vi "HGF_DSCVarManagerTask.vi"(1 "Task Trigger":refnum<class>, 2 "Task Destination":refnum<class>, 3 "Task Exception Event":refnum<class>, 5 "error in (no error)":errorcluster, 8 "timeout in ms (10000)":i32=10000, 9 "object/ProcessName":string) -> (14 "VarManager TaskLoop":refnum<class "HGF_TaskLoop.lvclass">, 16 "Task Trigger Event":refnum<class "HGF_Event.lvclass">, 17 "Task Destination Event":refnum<class "HGF_Event.lvclass">, 18 "ExceptionTriggerEvent":refnum<class "HGF_TriggeredEvent.lvclass">, 19 "error out":errorcluster)   [LabVIEW 2012, in "HGF_DSC.lvlib" / "HGF_DSCVarManager.lvclass"]
uses:
  HGF_DSCVarManager.lvclass
  HGF_BaseClasses/HGF_TriggeredEvent/HGF_TriggeredEvent.lvclass
  HGF_BaseClasses/HGF_Event/HGF_Event.lvclass
  HGF_BaseClasses/HGF_TaskLoop/HGF_TaskLoop.lvclass
  HGF_DSCFactory/HGF_DSCFactory.lvclass
  HGF_BaseClasses/HGF_Notifier/HGF_Notifier.lvclass
  HGF_BaseClasses/HGF_TaskOnce/HGF_TaskOnce.lvclass
  HGF_BaseClasses/HGF_ThreadTask/HGF_ThreadTask.lvclass
  HGF_BaseClasses/HGF_Factory/HGF_Factory.lvclass
  HGF_BaseClasses/HGF_Queue/HGF_Queue.lvclass
  HGF_BaseClasses/HGF_Timing/HGF_Timing.lvclass
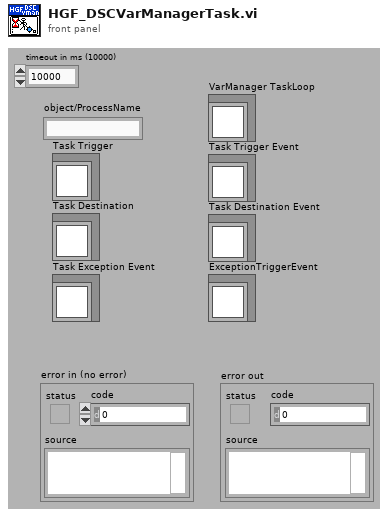
[diagram p1: front panel]
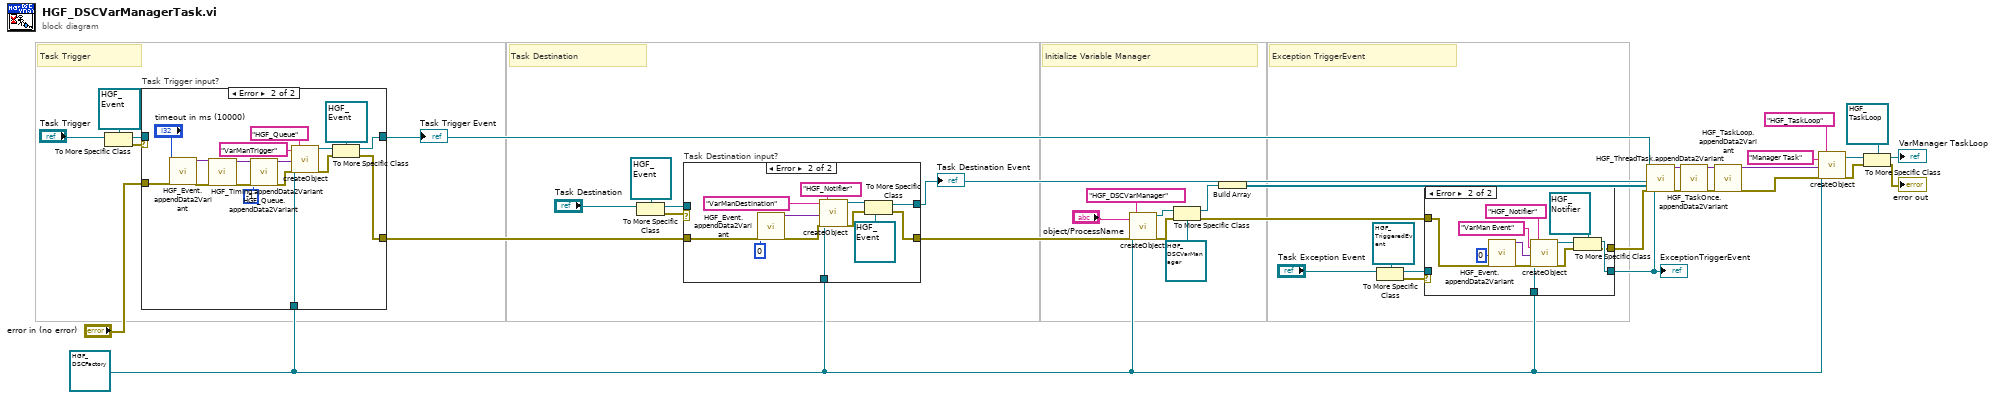
[diagram p0: block diagram]
diagram:
  w31 = refnum<class "HGF_DSCFactory.lvclass"> refnum ("DSC.lvlib:HGF_DSCFactory.lvclass")
  # "Exception TriggerEvent"
  # "Initialize Variable Manager"
  # "Task Destination"
  # "Task Trigger"
  n1 = To More Specific Class(target class=refnum<class "HGF_Event.lvclass"> refnum ("HGF_BaseClasses.lvlib:HGF_Event.lvclass"), reference="Task Trigger") -> (specific class reference=w29:refnum<class "HGF_Event.lvclass">, error out=w28:errorcluster)  [unwired: 1 in]
  n2 = case "Task Trigger input?" shown="Error" w28 {
    tunnel: w31 -> [_ w60]
    tunnel: [w43 w57] -> w30
    tunnel: [w42 w48] -> w35
    tunnel: "error in (no error)" -> [w42 w47]
    tunnel: w29 -> [w43 _]
    frame No Error {
    }
    frame Error {
      n3 = call "HGF_Event.appendData2Variant.vi"("timeout in ms (-1)"="timeout in ms (10000)", "error in (no error)"=w47) -> ("dup initData"=w50:variant, "error out"=w49:errorcluster)  [unwired: 16 in]
      n4 = call "HGF_Timing.appendData2Variant.vi"("initData"=w50, "error in (no error)"=w49) -> ("dup initData"=w53:variant, "error out"=w52:errorcluster)  [unwired: 16 in]
      n5 = call "HGF_Queue.appendData2Variant.vi"("initData"=w53, "maxQueueSize (-1)"=-1, "error in (no error)"=w52) -> ("dup initData"=w56:variant, "error out"=w55:errorcluster)  [unwired: 15 in]
      n6 = call "createObject.vi"("HGF_Factory"=w60, "objectName"="VarManTrigger", "initializationData"=w56, "error in (no error)"=w55, "className"="HGF_Queue") -> ("HGF_Object"=w59:refnum<class "HGF_Factory.lvclass">, "error out"=w58:errorcluster)  [unwired: 12 in, 1 out]
      n7 = To More Specific Class(target class=refnum<class "HGF_Event.lvclass"> refnum ("HGF_BaseClasses.lvlib:HGF_Event.lvclass"), reference=w59, error in=w58) -> (specific class reference=w57:refnum<class "HGF_Event.lvclass">, error out=w48:errorcluster)
    }
  }
  "Task Trigger Event" <- w30
  n8 = To More Specific Class(target class=refnum<class "HGF_Event.lvclass"> refnum ("HGF_BaseClasses.lvlib:HGF_Event.lvclass"), reference="Task Destination") -> (specific class reference=w36:refnum<class "HGF_Event.lvclass">, error out=w34:errorcluster)  [unwired: 1 in]
  n9 = case "Task Destination input?" shown="Error" w34 {
    tunnel: [w62 w71] -> w16
    tunnel: [w61 w70] -> w3
    tunnel: w35 -> [w61 w67]
    tunnel: w31 -> [_ w64]
    tunnel: w36 -> [w62 _]
    frame No Error {
    }
    frame Error {
      n10 = call "HGF_Event.appendData2Variant.vi"("timeout in ms (-1)"=0, "error in (no error)"=w67) -> ("dup initData"=w69:variant, "error out"=w68:errorcluster)  [unwired: 16 in]
      n11 = call "createObject.vi"("HGF_Factory"=w64, "objectName"="VarManDestination", "initializationData"=w69, "error in (no error)"=w68, "className"="HGF_Notifier") -> ("HGF_Object"=w73:refnum<class "HGF_Factory.lvclass">, "error out"=w72:errorcluster)  [unwired: 12 in, 1 out]
      n12 = To More Specific Class(target class=refnum<class "HGF_Event.lvclass"> refnum ("HGF_BaseClasses.lvlib:HGF_Event.lvclass"), reference=w73, error in=w72) -> (specific class reference=w71:refnum<class "HGF_Event.lvclass">, error out=w70:errorcluster)
    }
  }
  "Task Destination Event" <- w16
  n13 = call "createObject.vi"("HGF_Factory"=w31, "objectName"="object/ProcessName", "error in (no error)"=w3, "className"="HGF_DSCVarManager") -> ("HGF_Object"=w13:refnum<class "HGF_Factory.lvclass">, "error out"=w15:errorcluster)  [unwired: 13 in, 1 out]
  n14 = To More Specific Class(target class=refnum<class "HGF_DSCVarManager.lvclass"> refnum ("DSC.lvlib:HGF_DSCVarManager.lvclass"), reference=w13, error in=w15) -> (specific class reference=w14:refnum<class "HGF_DSCVarManager.lvclass">, error out=w18:errorcluster)
  n15 = Build Array(w14) -> (w12:refnum<class "HGF_DSCVarManager.lvclass">[])
  n16 = To More Specific Class(target class=refnum<class "HGF_TriggeredEvent.lvclass"> refnum ("HGF_BaseClasses.lvlib:HGF_TriggeredEvent.lvclass"), reference="Task Exception Event") -> (specific class reference=w39:refnum<class "HGF_TriggeredEvent.lvclass">, error out=w38:errorcluster)  [unwired: 1 in]
  n17 = case shown="Error" w38 {
    tunnel: [w76 w84] -> w40
    tunnel: [w75 w83] -> w17
    tunnel: w18 -> [w75 w82]
    tunnel: w31 -> [_ w77]
    tunnel: w39 -> [w76 _]
    frame No Error {
    }
    frame Error {
      n18 = call "HGF_Event.appendData2Variant.vi"("timeout in ms (-1)"=0, "error in (no error)"=w82) -> ("dup initData"=w80:variant, "error out"=w81:errorcluster)  [unwired: 16 in]
      n19 = call "createObject.vi"("HGF_Factory"=w77, "objectName"="VarMan Event", "initializationData"=w80, "error in (no error)"=w81, "className"="HGF_Notifier") -> ("HGF_Object"=w87:refnum<class "HGF_Factory.lvclass">, "error out"=w86:errorcluster)  [unwired: 12 in, 1 out]
      n20 = To More Specific Class(target class=refnum<class "HGF_Notifier.lvclass"> refnum ("HGF_BaseClasses.lvlib:HGF_Notifier.lvclass"), reference=w87, error in=w86) -> (specific class reference=w84:refnum<class "HGF_Notifier.lvclass">, error out=w83:errorcluster)
    }
  }
  "ExceptionTriggerEvent" <- w40
  n21 = call "HGF_ThreadTask.appendData2Variant.vi"("taskTrigger"=w30, "taskDestination"=w16, "objectArray"=w12, "error in (no error)"=w17, "exceptionEvent"=w40) -> ("dup initData"=w4:variant, "error out"=w10:errorcluster)  [unwired: 13 in]
  n22 = call "HGF_TaskOnce.appendData2Variant.vi"("initData"=w4, "error in (no error)"=w10) -> ("dup initData"=w5:variant, "error out"=w9:errorcluster)  [unwired: 16 in]
  n23 = call "HGF_TaskLoop.appendData2Variant.vi"("initData"=w5, "error in (no error)"=w9) -> ("dup initData"=w23:variant, "error out"=w22:errorcluster)  [unwired: 16 in]
  n24 = call "createObject.vi"("HGF_Factory"=w31, "objectName"="Manager Task", "initializationData"=w23, "error in (no error)"=w22, "className"="HGF_TaskLoop") -> ("HGF_Object"=w8:refnum<class "HGF_Factory.lvclass">, "error out"=w7:errorcluster)  [unwired: 12 in, 1 out]
  n25 = To More Specific Class(target class=refnum<class "HGF_TaskLoop.lvclass"> refnum ("HGF_BaseClasses.lvlib:HGF_TaskLoop.lvclass"), reference=w8, error in=w7) -> (specific class reference=→"VarManager TaskLoop":refnum<class "HGF_TaskLoop.lvclass">, error out=→"error out":errorcluster)
